vi "Test Module.vi"(8 "error in":errorcluster, 10 "TestCase in":refnum<class "Scan Engine Scripting API Modules.lvclass">, 11 "module test in":refnum<class "Module Test.lvclass">) -> (0 "error out":errorcluster, 2 "TestCase out":refnum<class "Scan Engine Scripting API Modules.lvclass">, 3 "module test out":refnum<class "Module Test.lvclass">)   [LabVIEW 2020, in "Module Test.lvclass"]
uses:
  Module Test.lvclass
  Scan Engine Scripting API Modules.lvclass
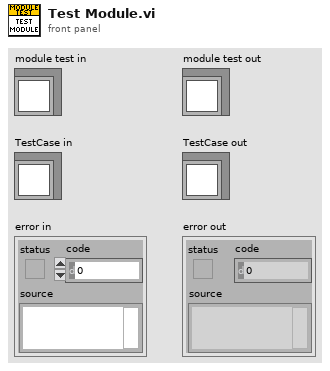
[diagram p1: front panel]
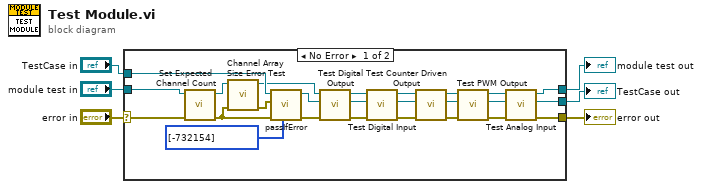
[diagram p0: block diagram]
diagram:
  n1 = case shown="No Error" "error in" {
    selector: "error in" -> [w28 w34]
    tunnel: [w13 w34] -> w5
    tunnel: [w15 w33] -> w3
    tunnel: "module test in" -> [w29 w33]
    tunnel: "TestCase in" -> [w30 w32]
    tunnel: [w17 w32] -> w1
    frame No Error {
      n2 = call-dynamic "Set Expected Channel Count.vi"("error in"=w28, "module test in"=w29) -> ("error out"=w20:errorcluster, "module test out"=w27:refnum<class "Module Test.lvclass">)  [unwired: 8 in]
      n3 = call-dynamic "Channel Array Size Error Test.vi"("error in"=w20, "module test in"=w27) -> ("error out"=w31:errorcluster, "module test out"=w26:refnum<class "Module Test.lvclass">)  [unwired: 8 in]
      n4 = call-dynamic "passIfError.vi"("passing error codes (default = any error code)"=i32[] [-732154], "error in (no error)"=w20, "error"=w31, "TestCase in"=w30) -> ("error out"=w24:errorcluster, "TestCase out"=w25:refnum<class "Scan Engine Scripting API Modules.lvclass">)  [unwired: 6 in]
      n5 = call-dynamic "Test Digital Output.vi"("error in"=w24, "TestCase in"=w25, "module test in"=w26) -> ("error out"=w11:errorcluster, "TestCase out"=w8:refnum<class "Scan Engine Scripting API Modules.lvclass">, "module test out"=w12:refnum<class "Module Test.lvclass">)  [unwired: 6 in]
      n6 = call-dynamic "Test Digital Input.vi"("error in"=w11, "TestCase in"=w8, "module test in"=w12) -> ("error out"=w9:errorcluster, "TestCase out"=w7:refnum<class "Scan Engine Scripting API Modules.lvclass">, "module test out"=w10:refnum<class "Module Test.lvclass">)  [unwired: 6 in]
      n7 = call-dynamic "Test Counter Driven Output.vi"("error in"=w9, "TestCase in"=w7, "module test in"=w10) -> ("error out"=w23:errorcluster, "TestCase out"=w22:refnum<class "Scan Engine Scripting API Modules.lvclass">, "module test out"=w21:refnum<class "Module Test.lvclass">)  [unwired: 6 in]
      n8 = call-dynamic "Test PWM Output.vi"("error in"=w23, "TestCase in"=w22, "module test in"=w21) -> ("error out"=w14:errorcluster, "TestCase out"=w18:refnum<class "Scan Engine Scripting API Modules.lvclass">, "module test out"=w16:refnum<class "Module Test.lvclass">)  [unwired: 6 in]
      n9 = call-dynamic "Test Analog Input.vi"("error in"=w14, "TestCase in"=w18, "module test in"=w16) -> ("error out"=w13:errorcluster, "TestCase out"=w17:refnum<class "Scan Engine Scripting API Modules.lvclass">, "module test out"=w15:refnum<class "Module Test.lvclass">)  [unwired: 6 in]
    }
    frame Error {
    }
  }
  "error out" <- w5
  "module test out" <- w3
  "TestCase out" <- w1
